vi "Example - Cluster.vi"() -> ()   [LabVIEW 2020]
uses:
  EquipmentVariant/Type Enum.ctl
  EquipmentVariant/EquipmentVariant.lvclass
  Robot/Robot.lvclass
  Pump/Pump.lvclass
panel:
  out "Pump 4":refnum<class "Pump.lvclass">
  out "Robot 3":refnum<class "Robot.lvclass">
  out "Pump":refnum<class "Pump.lvclass">
  out "Robot 2":refnum<class "Robot.lvclass">
  out "Pump 2":refnum<class "Pump.lvclass">
  out "Robot":refnum<class "Robot.lvclass">
  out "coerced 3":cluster{"Type":T1, "Variant":variant}
  out "coerced 2":cluster{"Type":T1, "Variant":variant}
  out "coerced 1":cluster{"Type":T1, "Variant":variant}
  out "Robot":refnum<class "Robot.lvclass">
  out "Pump":refnum<class "Pump.lvclass">
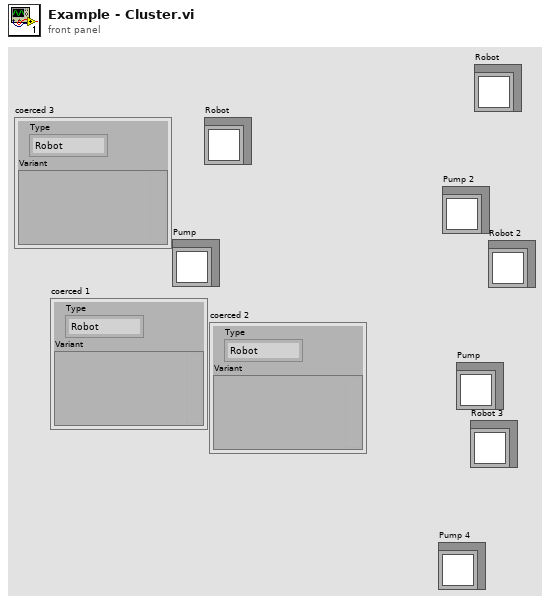
[diagram p1: front panel]
types:
  T1 = typedef "EquipmentVariant.lvclass/Type Enum.ctl" = enum16{"Robot", "Pump", "Instrument"}
  T2 = cluster{"Type":T1, "Robot.lvclass":refnum<class "Robot.lvclass">}
  T3 = cluster{"Type":T1, "Pump.lvclass":refnum<class "Pump.lvclass">}
  T4 = cluster{"Type":T1, "Instrument":refnum<visa-resource-name>}
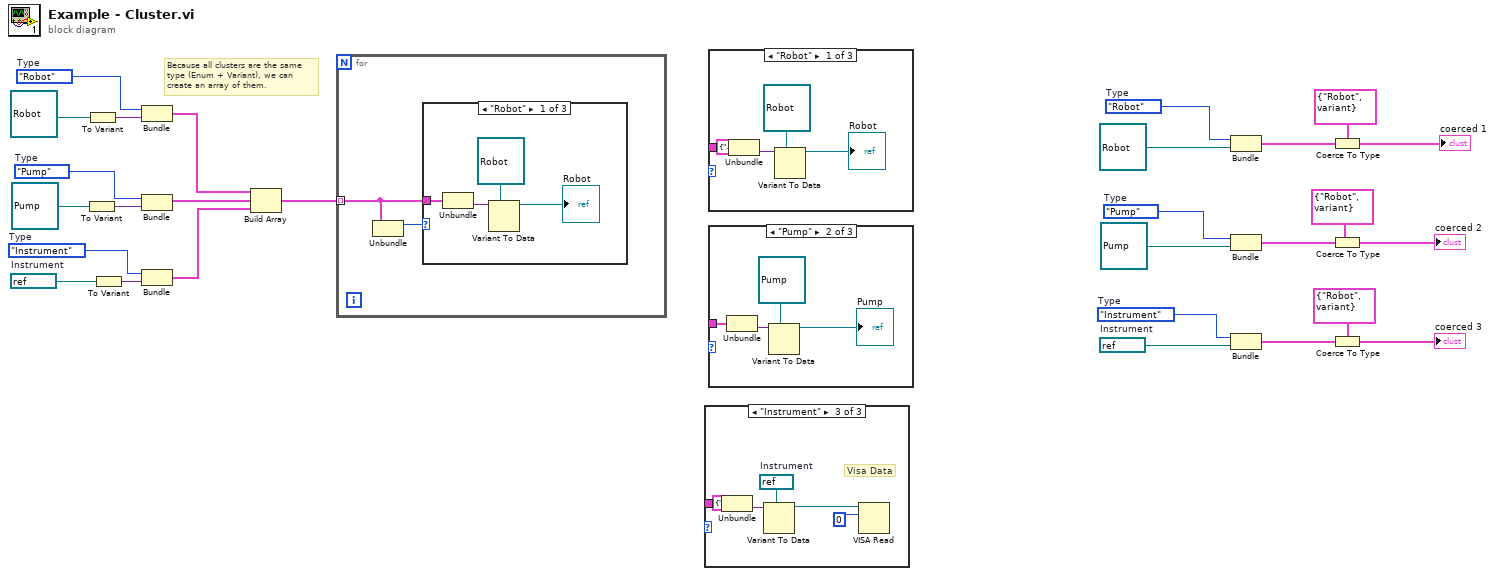
[diagram p0: block diagram]
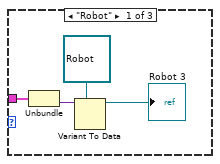
[diagram p2: hidden frame]
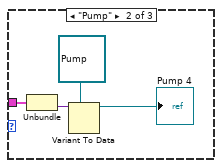
[diagram p3: hidden frame]
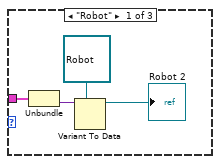
[diagram p4: hidden frame]
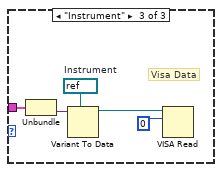
[diagram p5: hidden frame]
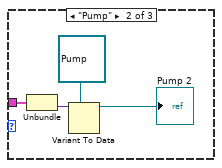
[diagram p6: hidden frame]
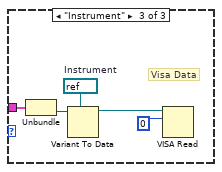
[diagram p7: hidden frame]
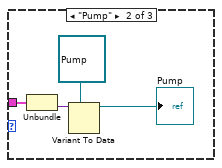
[diagram p8: hidden frame]
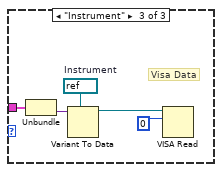
[diagram p9: hidden frame]
diagram:
  w15 = Type_Enum."Instrument"  # Type
  w14 = Type_Enum."Pump"  # Type
  w13 = Type_Enum."Robot"  # Type
  w17 = refnum<visa-resource-name> "abc"  # Instrument
  w28 = Type_Enum."Instrument"  # Type
  w29 = Type_Enum."Pump"  # Type
  w30 = Type_Enum."Robot"  # Type
  w21 = refnum<visa-resource-name> "abc"  # Instrument
  # "Because all clusters are the same type (Enum + Variant), we can create an array of them."
  n1 = To Variant(anything=refnum<class "Pump.lvclass"> refnum ("Pump.lvclass")) -> (Variant=w23:variant)
  n2 = To Variant(anything=refnum<class "Robot.lvclass"> refnum ("Robot.lvclass")) -> (Variant=w31:variant)
  n3 = To Variant(anything=w21) -> (Variant=w22:variant)
  n4 = Bundle("Type"=w30, "Variant"=w31) -> (w24:cluster{"Type":T1, "Variant":variant})  [unwired: 1 in]
  n5 = Bundle("Type"=w29, "Variant"=w23) -> (w27:cluster{"Type":T1, "Variant":variant})  [unwired: 1 in]
  n6 = Bundle("Type"=w28, "Variant"=w22) -> (w26:cluster{"Type":T1, "Variant":variant})  [unwired: 1 in]
  n7 = Build Array(w24, w27, w26) -> (w25:cluster{"Type":T1, "Variant":variant}[])
  n8 = for {
    tunnel: w25 -> [w33] mode=indexing
    n9 = Unbundle(w33) -> ("Type"=w32:T1)  [unwired: 1 out]
    n10 = case shown="\"Robot\"" w32 {
      tunnel: w33 -> [w37 w41 w44]
      frame "Robot" {
        n11 = Unbundle(w37) -> ("Variant"=w36:variant)  [unwired: 1 out]
        n12 = Variant To Data(type=refnum<class "Robot.lvclass"> refnum ("Robot.lvclass"), Variant=w36) -> (data=→"Robot":refnum<class "Robot.lvclass">)  [unwired: 1 in, 1 out]
      }
      frame "Pump" {
        n13 = Unbundle(w41) -> ("Variant"=w40:variant)  [unwired: 1 out]
        n14 = Variant To Data(type=refnum<class "Pump.lvclass"> refnum ("Pump.lvclass"), Variant=w40) -> (data=→"Pump":refnum<class "Pump.lvclass">)  [unwired: 1 in, 1 out]
      }
      frame "Instrument" {
        w45 = refnum<visa-resource-name> refnum  # Instrument
        # "Visa Data"
        n15 = Unbundle(w44) -> ("Variant"=w43:variant)  [unwired: 1 out]
        n16 = Variant To Data(type=w45, Variant=w43) -> (data=w42:refnum<visa-resource-name>)  [unwired: 1 in, 1 out]
        n17 = VISA Read(VISA resource name=w42, byte count=u32 0) -> ()  [unwired: 1 in, 4 out]
      }
    }
  }
  n18 = case shown="\"Instrument\"" {
    selector: _ -> [_ _ _]
    tunnel: cluster{"Type":T1, "Variant":variant} {"Type"=enum."Robot", "Variant"=variant} ("output cluster") -> [w50 w54 w57]
    frame "Robot" {
      n19 = Unbundle(w50) -> ("Variant"=w49:variant)  [unwired: 1 out]
      n20 = Variant To Data(type=refnum<class "Robot.lvclass"> refnum ("Robot.lvclass"), Variant=w49) -> (data=→"Robot 3":refnum<class "Robot.lvclass">)  [unwired: 1 in, 1 out]
    }
    frame "Pump" {
      n21 = Unbundle(w54) -> ("Variant"=w53:variant)  [unwired: 1 out]
      n22 = Variant To Data(type=refnum<class "Pump.lvclass"> refnum ("Pump.lvclass"), Variant=w53) -> (data=→"Pump 4":refnum<class "Pump.lvclass">)  [unwired: 1 in, 1 out]
    }
    frame "Instrument" {
      w58 = refnum<visa-resource-name> refnum  # Instrument
      # "Visa Data"
      n23 = Unbundle(w57) -> ("Variant"=w56:variant)  [unwired: 1 out]
      n24 = Variant To Data(type=w58, Variant=w56) -> (data=w55:refnum<visa-resource-name>)  [unwired: 1 in, 1 out]
      n25 = VISA Read(VISA resource name=w55, byte count=u32 0) -> ()  [unwired: 1 in, 4 out]
    }
  }
  n26 = case shown="\"Robot\"" {
    selector: _ -> [_ _ _]
    tunnel: cluster{"Type":T1, "Variant":variant} {"Type"=enum."Robot", "Variant"=variant} ("output cluster") -> [w63 w67 w70]
    frame "Robot" {
      n27 = Unbundle(w63) -> ("Variant"=w62:variant)  [unwired: 1 out]
      n28 = Variant To Data(type=refnum<class "Robot.lvclass"> refnum ("Robot.lvclass"), Variant=w62) -> (data=→"Robot":refnum<class "Robot.lvclass">)  [unwired: 1 in, 1 out]
    }
    frame "Pump" {
      n29 = Unbundle(w67) -> ("Variant"=w66:variant)  [unwired: 1 out]
      n30 = Variant To Data(type=refnum<class "Pump.lvclass"> refnum ("Pump.lvclass"), Variant=w66) -> (data=→"Pump 2":refnum<class "Pump.lvclass">)  [unwired: 1 in, 1 out]
    }
    frame "Instrument" {
      w71 = refnum<visa-resource-name> refnum  # Instrument
      # "Visa Data"
      n31 = Unbundle(w70) -> ("Variant"=w69:variant)  [unwired: 1 out]
      n32 = Variant To Data(type=w71, Variant=w69) -> (data=w68:refnum<visa-resource-name>)  [unwired: 1 in, 1 out]
      n33 = VISA Read(VISA resource name=w68, byte count=u32 0) -> ()  [unwired: 1 in, 4 out]
    }
  }
  n34 = case shown="\"Pump\"" {
    selector: _ -> [_ _ _]
    tunnel: cluster{"Type":T1, "Variant":variant} {"Type"=enum."Robot", "Variant"=variant} ("output cluster") -> [w76 w80 w83]
    frame "Robot" {
      n35 = Unbundle(w76) -> ("Variant"=w75:variant)  [unwired: 1 out]
      n36 = Variant To Data(type=refnum<class "Robot.lvclass"> refnum ("Robot.lvclass"), Variant=w75) -> (data=→"Robot 2":refnum<class "Robot.lvclass">)  [unwired: 1 in, 1 out]
    }
    frame "Pump" {
      n37 = Unbundle(w80) -> ("Variant"=w79:variant)  [unwired: 1 out]
      n38 = Variant To Data(type=refnum<class "Pump.lvclass"> refnum ("Pump.lvclass"), Variant=w79) -> (data=→"Pump":refnum<class "Pump.lvclass">)  [unwired: 1 in, 1 out]
    }
    frame "Instrument" {
      w84 = refnum<visa-resource-name> refnum  # Instrument
      # "Visa Data"
      n39 = Unbundle(w83) -> ("Variant"=w82:variant)  [unwired: 1 out]
      n40 = Variant To Data(type=w84, Variant=w82) -> (data=w81:refnum<visa-resource-name>)  [unwired: 1 in, 1 out]
      n41 = VISA Read(VISA resource name=w81, byte count=u32 0) -> ()  [unwired: 1 in, 4 out]
    }
  }
  n42 = Bundle("Type"=w13, "Robot.lvclass"=refnum<class "Robot.lvclass"> refnum) -> (w11:T2)  [unwired: 1 in]
  n43 = Bundle("Type"=w14, "Pump.lvclass"=refnum<class "Pump.lvclass"> refnum) -> (w9:T3)  [unwired: 1 in]
  n44 = Bundle("Type"=w15, "Instrument"=w17) -> (w7:T4)  [unwired: 1 in]
  n45 = Coerce To Type(0:w11, 1:cluster{"Type":T1, "Variant":variant} {"Type"=enum."Robot", "Variant"=variant} ("output cluster")) -> (2:→"coerced 1":cluster{"Type":T1, "Variant":variant})
  n46 = Coerce To Type(0:w9, 1:cluster{"Type":T1, "Variant":variant} {"Type"=enum."Robot", "Variant"=variant} ("output cluster")) -> (2:→"coerced 2":cluster{"Type":T1, "Variant":variant})
  n47 = Coerce To Type(0:w7, 1:cluster{"Type":T1, "Variant":variant} {"Type"=enum."Robot", "Variant"=variant} ("output cluster")) -> (2:→"coerced 3":cluster{"Type":T1, "Variant":variant})
